vi "AsyncSystemExec.vi"(8 "error in (no error)":errorcluster, 9 "Caller Events":T1, 10 "Working directory":path, 11 "Command":string) -> (0 "error out":errorcluster, 2 "Standard Error":string, 3 "Standard Out":string)   [LabVIEW 2018, in "async-system-exec.lvlib"]
uses:
  async-system-exec.lvlib
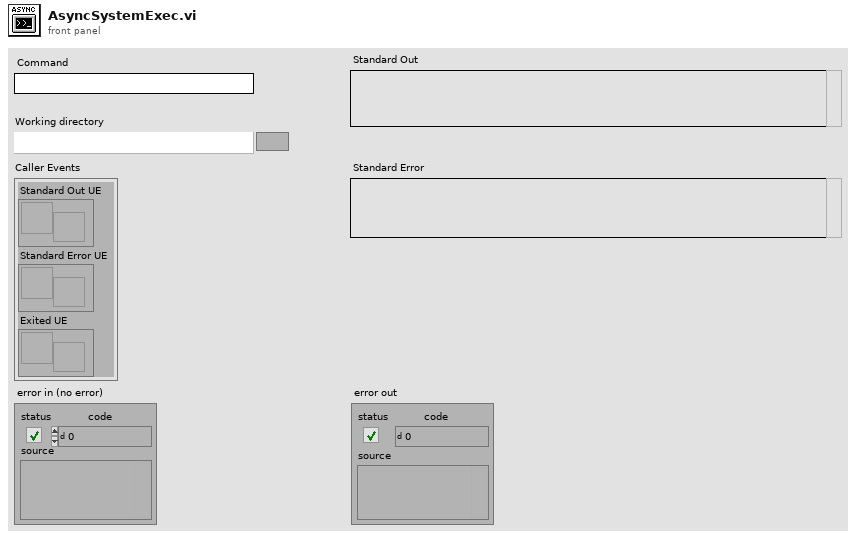
[diagram p1: front panel]
types:
  T1 = cluster{"Standard Out UE":refnum<user-event>, "Standard Error UE":refnum<user-event>, "Exited UE":refnum<user-event>}
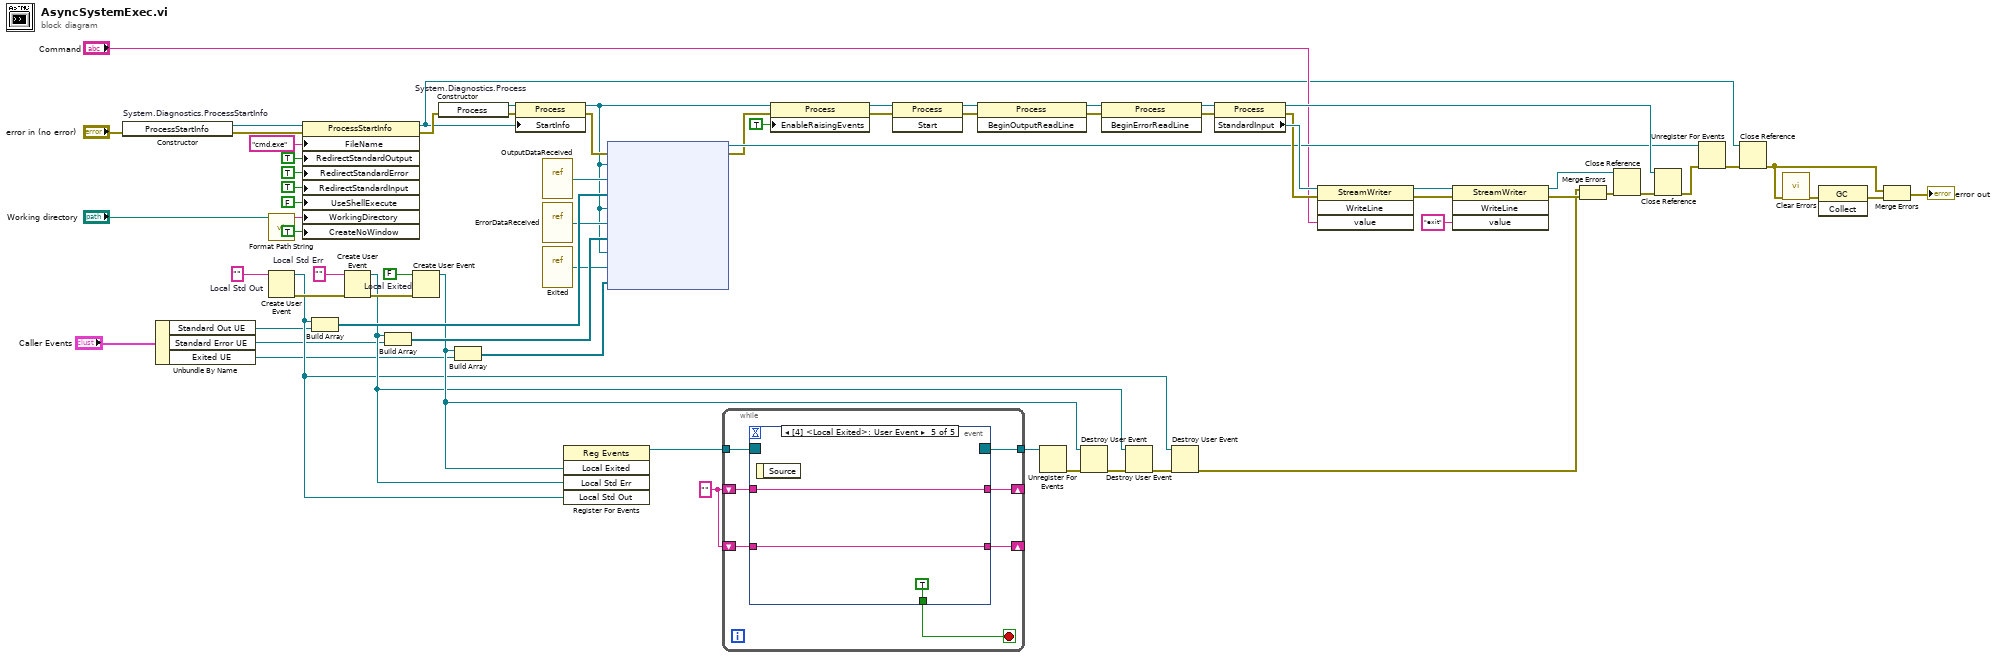
[diagram p0: block diagram]
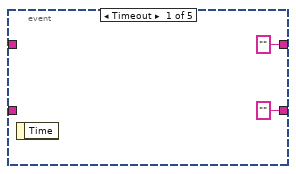
[diagram p2: hidden frame]
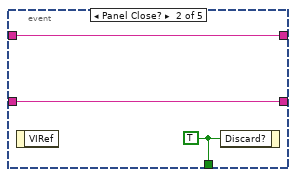
[diagram p3: hidden frame]
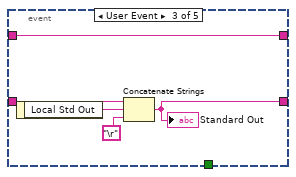
[diagram p4: hidden frame]
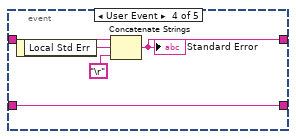
[diagram p5: hidden frame]
diagram:
  w5 = ""
  w24 = FALSE  # Local Exited
  w25 = ""  # Local Std Err
  w26 = ""  # Local Std Out
  n1 = constructor on="System.Diagnostics.ProcessStartInfo" class="ProcessStartInfo"(error in="error in (no error)") -> (reference out=w69:refnum<k24>, error out=w68:errorcluster)  [unwired: 2 in, 1 out]
  n2 = Unbundle By Name("Caller Events") -> ("Standard Out UE"=w3:refnum<user-event>, "Standard Error UE"=w2:refnum<user-event>, "Exited UE"=w1:refnum<user-event>)
  n3 = call "Format Path String.vi"("Path in"="Working directory") -> ("String out"=w61:string)  [unwired: 10 in]
  n4 = Create User Event(user event datatype=w26) -> (user event=w10:refnum<user-event>, error out=w23:errorcluster)  [unwired: 1 in]
  n5 = property class="ProcessStartInfo"(reference=w69, error in=w68, "FileName"="cmd.exe", "RedirectStandardOutput"=TRUE, "RedirectStandardError"=TRUE, "RedirectStandardInput"=TRUE, "UseShellExecute"=FALSE, "WorkingDirectory"=w61, "CreateNoWindow"=TRUE) -> (reference out=w31:refnum<k24>, error out=w57:errorcluster)
  n6 = Build Array(w10, w3) -> (w19:refnum<user-event>[])
  n7 = Create User Event(user event datatype=w25, error in=w23) -> (user event=w11:refnum<user-event>, error out=w22:errorcluster)
  n8 = Build Array(w11, w2) -> (w20:refnum<user-event>[])
  n9 = Create User Event(user event datatype=w24, error in=w22) -> (user event=w12:refnum<user-event>)  [unwired: 1 out]
  n10 = constructor on="System.Diagnostics.Process" class="Process"(error in=w57) -> (reference out=w58:refnum<k24>, error out=w59:errorcluster)  [unwired: 2 in, 1 out]
  n11 = Build Array(w12, w1) -> (w21:refnum<user-event>[])
  n12 = property class="Process"(reference=w58, error in=w59, "StartInfo"=w31) -> (reference out=w6:refnum<k24>, error out=w56:errorcluster)
  n13 = vi-ref "OutputDataReceived.vi"() -> ("vi reference"=w9:refnum<vi>)
  n14 = vi-ref "ErrorDataReceived.vi"() -> ("vi reference"=w8:refnum<vi>)
  n15 = vi-ref "Exited.vi"() -> ("vi reference"=w7:refnum<vi>)
  n16 = register-events(w12, w11, w10) -> (reference out=w18:refnum<event-registration>)  [unwired: 2 in, 1 out]
  n17 = node(w56, w6, w9, w19, w6, w8, w20, w6, w7, w21) -> (w33:refnum<k27>, w30:errorcluster)  [unwired: 1 in]
  n18 = while {
    tunnel: w18 -> [w76]
    tunnel: [w75] -> w17
    shift-right: [w73] -> _
    shift-left: w5 -> [w74]
    shift-right: [w72] -> _
    shift-left: w5 -> [w71]
    stop <- w77 stop-if-true
    n19 = event shown="[4] <Local Exited>: User Event" {
      selector: w76 -> [_ _ _ _ _]
      dyn-events: [_ _ _ _ _] -> w75
      timeout: _ -> [_ _ _ _ _]
      tunnel: [_ w82 _ _ TRUE] -> w77
      tunnel: w74 -> [_ w81 w86 w92 w95]
      tunnel: ["" w81 w84 w92 w95] -> w73
      tunnel: ["" w80 w83 w88 w93] -> w72
      tunnel: w71 -> [_ w80 w83 w90 w93]
      event Timeout {
        n20 = event-data() -> ()  [unwired: 1 in, 1 out]
      }
      event Panel Close? {
        w82 = TRUE
        n21 = event-data() -> ()  [unwired: 1 in, 1 out]
        n22 = event-data("Discard?"=w82) -> ()  [unwired: 1 in, 1 out]
      }
      event User Event {
        n23 = event-data() -> ("Local Std Out"=w85:string)  [unwired: 1 in]
        n24 = Concatenate Strings(w86, w85, "\r") -> (w84:string)
        "Standard Out" <- w84
      }
      event User Event {
        n25 = event-data() -> ("Local Std Err"=w89:string)  [unwired: 1 in]
        n26 = Concatenate Strings(w90, w89, "\r") -> (w88:string)
        "Standard Error" <- w88
      }
      event User Event {
        n27 = event-data() -> ()  [unwired: 1 in, 1 out]
      }
    }
  }
  n28 = property class="Process"(reference=w6, error in=w30, "EnableRaisingEvents"=TRUE) -> (reference out=w53:refnum<k24>, error out=w54:errorcluster)
  n29 = invoke class="Process" method="Start"(reference=w53, error in=w54) -> (reference out=w51:refnum<k24>, error out=w52:errorcluster)  [unwired: 1 in, 1 out]
  n30 = invoke class="Process" method="BeginOutputReadLine"(reference=w51, error in=w52) -> (reference out=w49:refnum<k24>, error out=w50:errorcluster)  [unwired: 1 in, 1 out]
  n31 = Unregister For Events(event registration refnum=w17) -> (error out=w16:errorcluster)  [unwired: 1 in]
  n32 = Destroy User Event(user event=w12, error in=w16) -> (error out=w14:errorcluster)
  n33 = invoke class="Process" method="BeginErrorReadLine"(reference=w49, error in=w50) -> (reference out=w48:refnum<k24>, error out=w47:errorcluster)  [unwired: 1 in, 1 out]
  n34 = Destroy User Event(user event=w11, error in=w14) -> (error out=w13:errorcluster)
  n35 = Destroy User Event(user event=w10, error in=w13) -> (error out=w15:errorcluster)
  n36 = property class="Process"(reference=w48, error in=w47) -> (reference out=w38:refnum<k24>, error out=w43:errorcluster, "StandardInput"=w46:refnum<k24>)
  n37 = invoke class="StreamWriter" method="WriteLine"(reference=w46, error in=w43, "value"="Command") -> (reference out=w45:refnum<k24>, error out=w44:errorcluster)  [unwired: 1 in, 2 out]
  n38 = invoke class="StreamWriter" method="WriteLine"(reference=w45, error in=w44, "value"="exit") -> (reference out=w40:refnum<k24>, error out=w41:errorcluster)  [unwired: 1 in, 2 out]
  n39 = Merge Errors(w15, w41) -> (w35:errorcluster)
  n40 = Close Reference(reference=w40, error in (no error)=w35) -> (error out=w39:errorcluster)
  n41 = Close Reference(reference=w38, error in (no error)=w39) -> (error out=w37:errorcluster)
  n42 = Unregister For Events(event registration refnum=w33, error in=w37) -> (error out=w36:errorcluster)
  n43 = Close Reference(reference=w31, error in (no error)=w36) -> (error out=w27:errorcluster)
  n44 = call <vilib>:"Clear Errors.vi"("error in (no error)"=w27) -> ("error out"=w34:errorcluster)  [unwired: 5 in, 1 out]
  n45 = invoke class="GC" method="Collect"(error in=w34) -> (error out=w29:errorcluster)  [unwired: 2 in, 2 out]
  n46 = Merge Errors(w27, w29) -> (→"error out":errorcluster)
